vi "Experiment 1.VI"() -> ()   [LabVIEW 2017]
panel:
  in  "stop":bool
  out "Tank":dbl(slide) scale=0.0..10.0
  in  "Slide":dbl(slide) scale=0.0..10.0
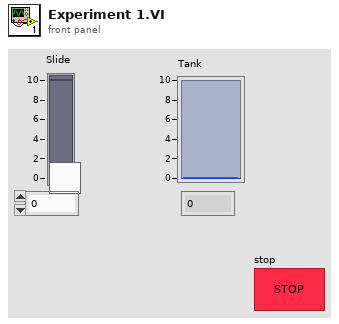
[diagram p1: front panel]
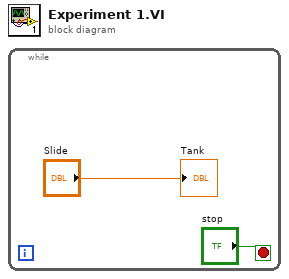
[diagram p0: block diagram]
diagram:
  n1 = while {
    stop <- "stop" stop-if-true
    "Tank" <- "Slide"
  }
